vi "getRandomLed.vi"(8 "error in (no error)":errorcluster, 11 "Simon_Engine in":refnum<class "Simon_Engine.lvclass">) -> (0 "error out":errorcluster, 3 "Simon_Engine out":refnum<class "Simon_Engine.lvclass">)   [LabVIEW 2019, in "Simon_Engine.lvclass"]
doc: "Chooses one of the LED randomly."
uses:
  Simon_Engine.lvclass
  Simon_Engine.lvclass/Simon_Engine.ctl
  <vilib>/numeric/Random Number (Range) U64.vi
  <vilib>/numeric/sub_Random U32.vi
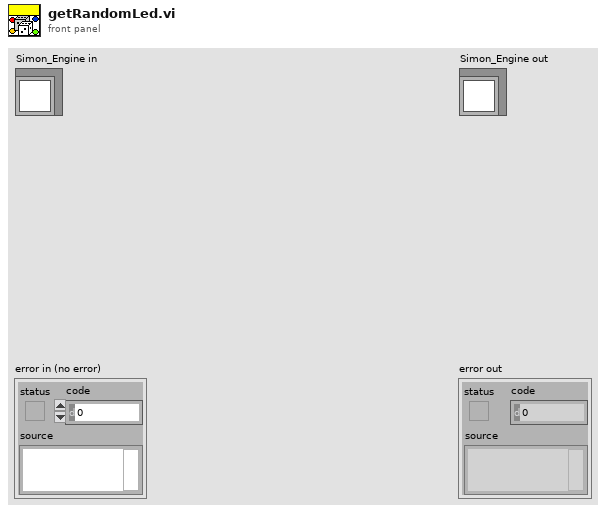
[diagram p1: front panel]
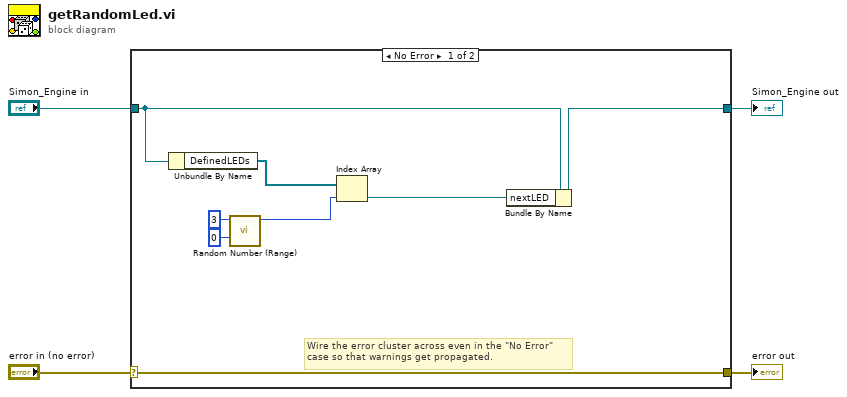
[diagram p0: block diagram]
diagram:
  n1 = case shown="No Error" "error in (no error)" {
    selector: "error in (no error)" -> [w12 w14]
    tunnel: [w12 w14] -> w3
    tunnel: [w6 w13] -> w1
    tunnel: "Simon_Engine in" -> [w11 w13]
    frame No Error {
      # "Wire the error cluster across even in the \"No Error\"\ncase so that warnings get propagated."
      n2 = Unbundle By Name(w11) -> ("DefinedLEDs"=w8:refnum<class "LED.lvclass">[])
      n3 = call-poly <vilib>:"Random Number (Range).vi"("lower bound (0)"=u64 0, "upper bound (100)"=u64 3) -> ("number"=w7:u64)  [unwired: 9 in]
      n4 = Index Array(array=w8, index=w7) -> (element=w5:refnum<class "LED.lvclass">)
      n5 = Bundle By Name(cluster=w11, "nextLED"=w5) -> (w6:refnum<class "Simon_Engine.lvclass">)
    }
    frame Error {
    }
  }
  "error out" <- w3
  "Simon_Engine out" <- w1
